vi "special Cx Deneme.vi"() -> ()   [LabVIEW 2013]
uses:
  Classes/OSSP_Problem.lvclass
  Classes/Scheduler.lvclass
panel:
  in  "Schedule 2":u16[](array[numeric])=[13, 14, 10, 7, 0, 3, 6, 11, 5, 12, 8, 9, 4, 2, 1, 15]
  in  "Schedule 1":u16[](array[numeric])=[12, 4, 13, 0, 14, 2, 7, 15, 9, 1, 6, 3, 11, 10, 5, 8]
  out "Array 2":i32[](array[numeric])
  out "Array":i32[](array[numeric])
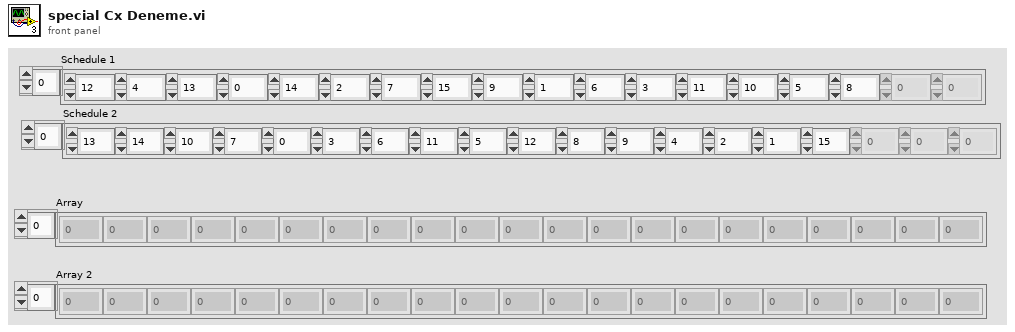
[diagram p1: front panel]
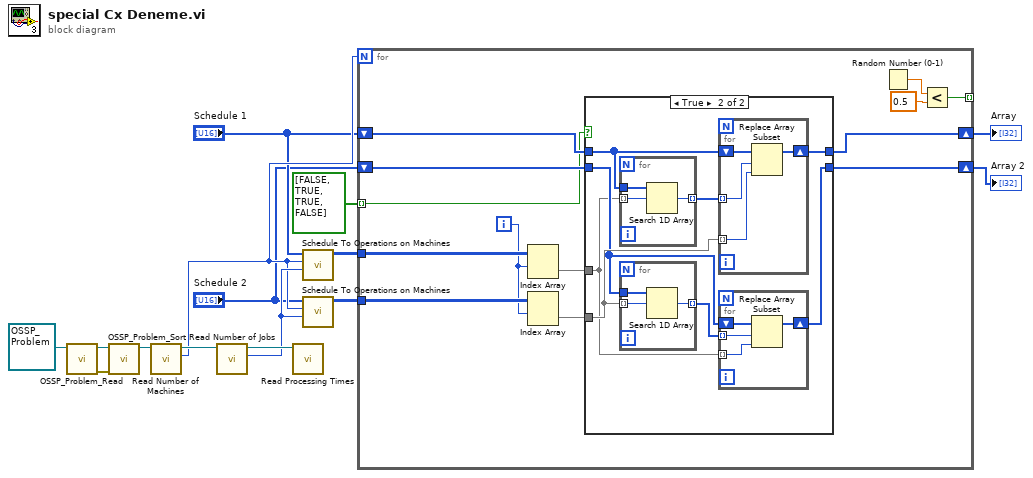
[diagram p0: block diagram]
diagram:
  n1 = call "OSSP_Problem_Read.vi"("OSSP_Problem.lvclass In"=refnum<class "OSSP_Problem.lvclass"> refnum ("OSSP_Problem.lvclass")) -> ("error out"=w13:errorcluster, "OSSP_Problem.lvclass Out"=w14:refnum<class "OSSP_Problem.lvclass">)  [unwired: 9 in]
  n2 = call "OSSP_Problem_Sort.vi"("error in (no error)"=w13, "OSSP_Problem.lvclass In"=w14) -> ("OSSP_Problem.lvclass Out"=w12:refnum<class "OSSP_Problem.lvclass">)  [unwired: 8 in, 1 out]
  n3 = call "Read Number of Machines.vi"("OSSP_Problem in"=w12) -> ("Number of Machines"=w4:i32, "OSSP_Problem out"=w11:refnum<class "OSSP_Problem.lvclass">)  [unwired: 8 in, 1 out]
  n4 = call "Read Number of Jobs.vi"("OSSP_Problem in"=w11) -> ("Number of Jobs"=w7:i32, "OSSP_Problem out"=w10:refnum<class "OSSP_Problem.lvclass">)  [unwired: 8 in, 1 out]
  n5 = call "Read Processing Times.vi"("OSSP_Problem in"=w10) -> ()  [unwired: 8 in, 3 out]
  n6 = call "Schedule To Operations on Machines.vi"("Number of Jobs"=w7, "Number of Machines"=w4, "Schedule"="Schedule 1") -> ("Operations On Machines"=w9:i32[][])  [unwired: 8 in]
  n7 = call "Schedule To Operations on Machines.vi"("Number of Jobs"=w7, "Number of Machines"=w4, "Schedule"="Schedule 2") -> ("Operations On Machines"=w8:i32[][])  [unwired: 8 in]
  n8 = for {
    N: w4 -> [_]
    tunnel: w9 -> [w22]
    tunnel: w8 -> [w24]
    shift-right: [w19] -> w6
    shift-left: "Schedule 1" -> [w25]
    shift-right: [w18] -> w5
    shift-left: "Schedule 2" -> [w26]
    tunnel: [w17] -> _ mode=indexing
    tunnel: bool[] [FALSE, TRUE, TRUE, FALSE] ("Array 3") -> [w16] mode=indexing
    i -> [w21]
    n9 = Index Array(array=w22, index (row)=w21) -> (element=w20:i32[])  [unwired: 1 in]
    n10 = Index Array(array=w24, index (row)=w21) -> (element=w23:i32[])  [unwired: 1 in]
    n11 = case shown="True" w16 {
      tunnel: w26 -> [w29 w34]
      tunnel: w25 -> [w30 w37]
      tunnel: w23 -> [_ w35]
      tunnel: w20 -> [_ w32]
      tunnel: [w30 w36] -> w19
      tunnel: [w29 w31] -> w18
      frame False {
      }
      frame True {
        n12 = for {
          tunnel: w32 -> [w52] mode=indexing
          tunnel: w37 -> [w51]
          tunnel: [w50] -> w38 mode=indexing
          n13 = Search 1D Array(1D array=w51, element=w52) -> (index of element=w50:i32)  [unwired: 1 in]
        }
        n14 = for {
          tunnel: w35 -> [w45] mode=indexing
          tunnel: w34 -> [w44]
          tunnel: [w43] -> w33 mode=indexing
          n15 = Search 1D Array(1D array=w44, element=w45) -> (index of element=w43:i32)  [unwired: 1 in]
        }
        n16 = for {
          tunnel: w38 -> [w48] mode=indexing
          tunnel: w35 -> [w47] mode=indexing
          shift-right: [w46] -> w36
          shift-left: w37 -> [w49]
          n17 = Replace Array Subset(array=w49, new element=w47, index=w48) -> (w46:u16[])
        }
        n18 = for {
          tunnel: w33 -> [w41] mode=indexing
          tunnel: w32 -> [w40] mode=indexing
          shift-right: [w39] -> w31
          shift-left: w34 -> [w42]
          n19 = Replace Array Subset(array=w42, new element=w40, index=w41) -> (w39:u16[])
        }
      }
    }
    n20 = Random Number (0-1)() -> (number: 0 to 1=w27:dbl)
    n21 = Less?(x=w27, y=0.5) -> (x < y?=w17:bool)
  }
  "Array" <- w6
  "Array 2" <- w5
